vi "Watflow F4 Profile.vi"() -> ()   [LabVIEW 2010]
doc: "This VI creates a new ramping profile and runs it.\n\nNote: \n(1) It represents the <B>Main>Profiles</B> menu of the controller.\n(2) To setup sensor type run WLF4 Analog Input Setup Example.vi."
uses:
  SubVIs/Watflow F4/Watflow F4.lvlib
panel:
  in  "Stop":bool
  out "Temperature Chart":cluster{"Value":dbl, "Value":dbl}(graph)
  in  "Time (0; 0; 1)":i16[](array[numeric])=[0, 0, 1]
  in  "Set Point Channel 1 (75.0)":dbl=75.0 format="%.2f"
  in  "Profile Name (PROFILE1)":string="PROFILE1"
  in  "Unit Address (1)":u8=1
  in  "Instrument Resource Name":refnum<visa-resource-name>
  in  "error in (no error)":errorcluster
  # "© 2005 National Instruments.  ALL RIGHTS RESERVED."
  # "WATLOW F4 Series"
  # "Main > Profile > Create Profile > Start a Profile"
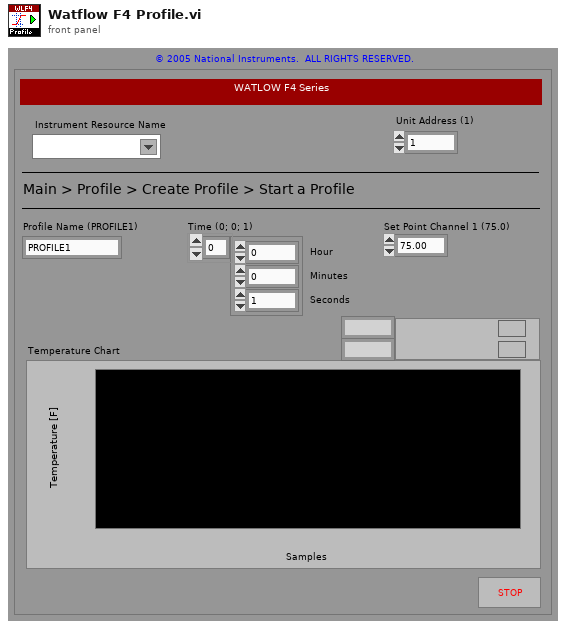
[diagram p1: front panel]
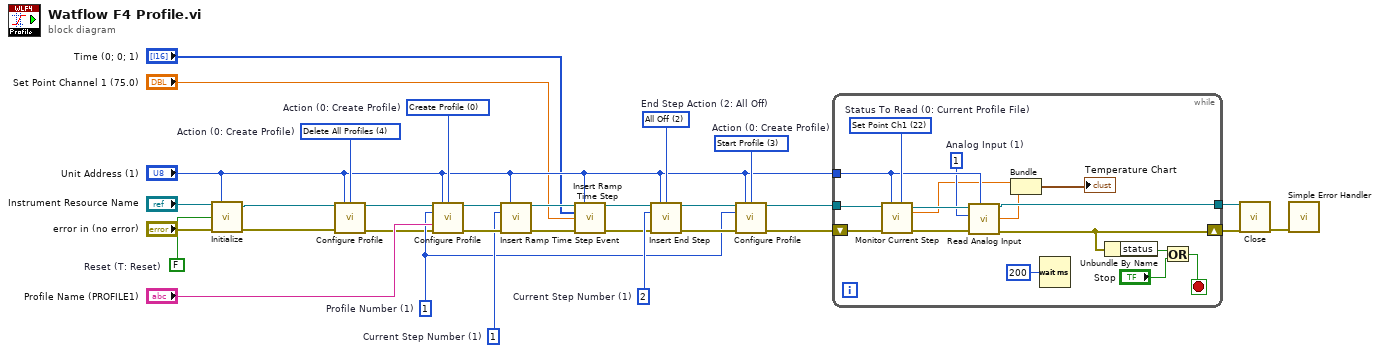
[diagram p0: block diagram]
diagram:
  w12 = u16 4 items=["Create Profile", "Delete Current Profile", "Delete Step", "Start Profile", "Delete All Profiles", "Rename Profile"]  # Action (0: Create Profile)
  w17 = i16 1  # Profile Number (1)
  w18 = u16 3 items=["Create Profile", "Delete Current Profile", "Delete Step", "Start Profile", "Delete All Profiles", "Rename Profile"]  # Action (0: Create Profile)
  w19 = u16 2 items=["Hold", "Control Off", "All Off", "Idle"]  # End Step Action (2: All Off)
  w20 = i16 2  # Current Step Number (1)
  w21 = i16 1  # Current Step Number (1)
  w27 = u16 0 items=["Create Profile", "Delete Current Profile", "Delete Step", "Start Profile", "Delete All Profiles", "Rename Profile"]  # Action (0: Create Profile)
  w28 = FALSE  # Reset (T: Reset)
  n1 = call "Initialize.vi"("VISA resource name"="Instrument Resource Name", "Unit Address (1)"="Unit Address (1)", "Reset (T: Reset)"=w28, "error in (no error)"="error in (no error)") -> ("VISA resource name out"=w10:refnum<visa-resource-name>, "error out"=w9:errorcluster)  [unwired: 10 in]
  n2 = call "Configure Profile.vi"("VISA resource name"=w10, "Unit Address (1)"="Unit Address (1)", "Action (0: Create Profile)"=w12, "error in (no error)"=w9) -> ("VISA resource name out"=w11:refnum<visa-resource-name>, "error out"=w8:errorcluster)  [unwired: 10 in]
  n3 = call "Configure Profile.vi"("VISA resource name"=w11, "Unit Address (1)"="Unit Address (1)", "Action (0: Create Profile)"=w27, "Profile Number (1)"=w17, "Profile Name (PROFILE1)"="Profile Name (PROFILE1)", "error in (no error)"=w8) -> ("VISA resource name out"=w24:refnum<visa-resource-name>, "error out"=w25:errorcluster)  [unwired: 8 in]
  n4 = call "Insert Ramp Time Step Event.vi"("VISA resource name"=w24, "Unit Address (1)"="Unit Address (1)", "Current Step Number (1)"=w21, "error in (no error)"=w25) -> ("VISA resource name out"=w7:refnum<visa-resource-name>, "error out"=w4:errorcluster)  [unwired: 10 in]
  n5 = call "Insert Ramp Time Step.vi"("VISA resource name"=w7, "Unit Address (1)"="Unit Address (1)", "Time (0; 0; 1)"="Time (0; 0; 1)", "Set Point Channel 1 (75.0)"="Set Point Channel 1 (75.0)", "error in (no error)"=w4) -> ("VISA resource name out"=w6:refnum<visa-resource-name>, "error out"=w5:errorcluster)  [unwired: 9 in]
  n6 = call "Insert End Step.vi"("VISA resource name"=w6, "Unit Address (1)"="Unit Address (1)", "End Step Action (2: All Off)"=w19, "Current Step Number (1)"=w20, "error in (no error)"=w5) -> ("VISA resource name out"=w22:refnum<visa-resource-name>, "error out"=w23:errorcluster)  [unwired: 9 in]
  n7 = call "Configure Profile.vi"("VISA resource name"=w22, "Unit Address (1)"="Unit Address (1)", "Action (0: Create Profile)"=w18, "Profile Number (1)"=w17, "error in (no error)"=w23) -> ("VISA resource name out"=w16:refnum<visa-resource-name>, "error out"=w14:errorcluster)  [unwired: 9 in]
  n8 = while {
    tunnel: w16 -> [w47]
    tunnel: [w41] -> w15
    tunnel: "Unit Address (1)" -> [w43]
    shift-right: [w37] -> w13
    shift-left: w14 -> [w38]
    stop <- w39 stop-if-true
    w35 = i16 1  # Analog Input (1)
    w46 = u16 22 items=["Current Profile File Number", "Current Profile Step Number", "Current Profile Step Type", "Profile Ramp Waiting", "Profile Waiting For Event 1", "Profile Waiting For Event 2", "Profile Waiting For Event 3", "Profile Waiting For Event 4", "Profile Waiting Analog Input 1", "Profile Waiting Analog Input 2", "Profile Waiting Analog Input 3", "Digital Output 1", "Digital Output 2", "Digital Output 3", "Digital Output 4", "Digital Output 5", "Digital Output 6", "Digital Output 7", "Digital Output 8", "Hours Remaining", "Minutes Remaining", "Seconds Remaining", "Set Point Ch1", "Set Point Ch2", "Ch1 PID Set", "Ch2 PID Set", "Last Jump Count", "Last Jump File", "Jump Step", "End Setpoint Ch1", "End Setpoint Ch2"]  # Status To Read (0: Current Profile File)
    n9 = call "Monitor Current Step.vi"("VISA resource name"=w47, "Unit Address (1)"=w43, "Status To Read (0: Current Profile File)"=w46, "error in (no error)"=w38) -> ("VISA resource name out"=w44:refnum<visa-resource-name>, "Value"=w34:dbl, "error out"=w45:errorcluster)  [unwired: 9 in]
    n10 = call "Read Analog Input.vi"("Unit Address (1)"=w43, "error in (no error)"=w45, "Analog Input (1)"=w35, "VISA resource name"=w44) -> ("error out"=w37:errorcluster, "Value"=w33:dbl, "VISA resource name out"=w41:refnum<visa-resource-name>)  [unwired: 5 in]
    n11 = Bundle("Value"=w34, "Value"=w33) -> (→"Temperature Chart":cluster{"Value":dbl, "Value":dbl})  [unwired: 1 in]
    n12 = Wait (ms)(milliseconds to wait=u32 200) -> ()  [unwired: 1 out]
    n13 = Unbundle By Name(w37) -> ("status"=w40:bool)
    n14 = Or(x=w40, y="Stop") -> (x .or. y?=w39:bool)
  }
  n15 = call "Close.vi"("VISA resource name"=w15, "error in (no error)"=w13) -> ("error out"=w29:errorcluster)  [unwired: 13 in]
  n16 = call <vilib>:"Simple Error Handler.vi"("error in (no error)"=w29) -> ()  [unwired: 4 in, 5 out]
